vi "сумматор(5-разрядный).vi"(2 "B":T2, 3 "A":T3) -> (0 "c":bool, 1 "R":T1)   [LabVIEW 2013]
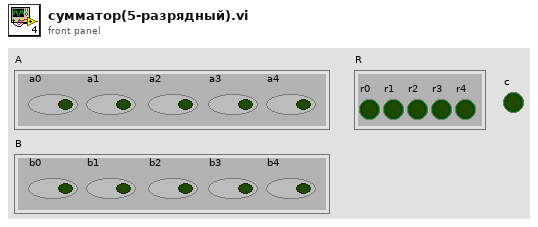
[diagram p1: front panel]
types:
  T1 = cluster{"r0":bool, "r1":bool, "r2":bool, "r3":bool, "r4":bool}
  T2 = cluster{"b0":bool, "b1":bool, "b2":bool, "b3":bool, "b4":bool}
  T3 = cluster{"a0":bool, "a1":bool, "a2":bool, "a3":bool, "a4":bool}
  T4 = cluster{"s":bool, "s":bool, "s":bool, "s":bool, "s":bool}
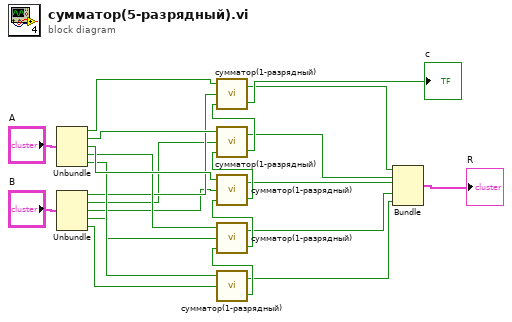
[diagram p0: block diagram]
diagram:
  n1 = Unbundle("A") -> ("a0"=w17:bool, "a1"=w16:bool, "a2"=w15:bool, "a3"=w14:bool, "a4"=w13:bool)
  n2 = Unbundle("B") -> ("b0"=w12:bool, "b1"=w11:bool, "b2"=w10:bool, "b3"=w9:bool, "b4"=w8:bool)
  n3 = call "сумматор(1-разрядный).vi"("b"=w8, "a"=w13) -> ("c"=w21:bool, "s"=w1:bool)  [unwired: 1 in]
  n4 = call "сумматор(1-разрядный).vi"("c-1"=w21, "b"=w9, "a"=w14) -> ("c"=w20:bool, "s"=w2:bool)
  n5 = call "сумматор(1-разрядный).vi"("c-1"=w20, "b"=w10, "a"=w15) -> ("c"=w19:bool, "s"=w3:bool)
  n6 = call "сумматор(1-разрядный).vi"("c-1"=w19, "b"=w11, "a"=w16) -> ("c"=w18:bool, "s"=w4:bool)
  n7 = call "сумматор(1-разрядный).vi"("c-1"=w18, "b"=w12, "a"=w17) -> ("c"=→"c":bool, "s"=w5:bool)
  n8 = Bundle("s"=w5, "s"=w4, "s"=w3, "s"=w2, "s"=w1) -> (→"R":T4)  [unwired: 1 in]
